vi "Set Random Colors.vi"(1 "Instrument Prop In":T1 {"Private"."Offset" format="%^_3e"; "Private"."Scale Factors" format="%^_3e"}) -> (0 "Instrument Prop Out":T1 {"Private"."Offset" format="%^_3e"; "Private"."Scale Factors" format="%^_3e"})   [LabVIEW 2019]
uses:
  Sub Controls/Instrument Properties.ctl
  Sub Controls/Public.ctl
  Sub Controls/Private.ctl
  Sub Controls/Instrument Ref.ctl
  Sub Controls/SystemCheckBox-resize.ctl
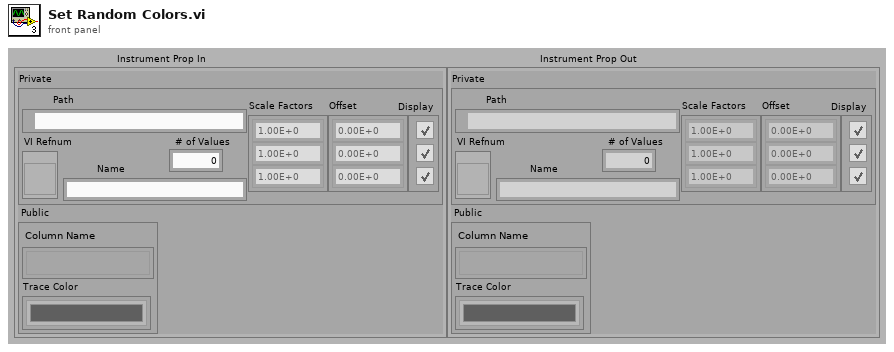
[diagram p1: front panel]
types:
  T1 = typedef "Instrument Properties.ctl" = cluster{"Public":T2, "Private":T3}
  T2 = typedef "Public.ctl" = cluster{"Column Name":string[], "Trace Color":u32[]}
  T3 = typedef "Private.ctl" = cluster{"Path":path, "VI Refnum":T4, "Name":string, "# of Values":i32, "Scale Factors":dbl[], "Display":T5[], "Offset":dbl[]}
  T4 = typedef "Instrument Ref.ctl" = refnum<vi>
  T5 = typedef "SystemCheckBox-resize.ctl" = bool
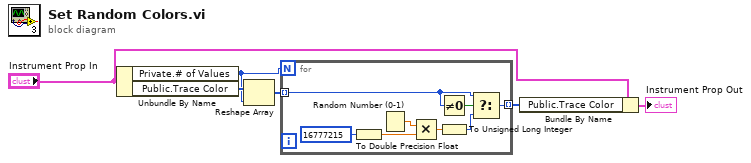
[diagram p0: block diagram]
diagram:
  n1 = Unbundle By Name("Instrument Prop In") -> ("Private.# of Values"=w1:i32, "Public.Trace Color"=w4:u32[])
  n2 = Reshape Array(w4, w1) -> (w2:u32[])
  n3 = for {
    N: w1 -> [_]
    tunnel: w2 -> [w10] mode=indexing
    tunnel: [w9] -> w3 mode=indexing
    n4 = To Double Precision Float(number=u32 16777215 ("y")) -> (double precision float=w7:dbl)
    n5 = Random Number (0-1)() -> (number: 0 to 1=w14:dbl)
    n6 = Multiply(x=w14, y=w7) -> (x*y=w12:dbl)
    n7 = Not Equal To 0?(x=w10) -> (x != 0?=w11:bool)
    n8 = To Unsigned Long Integer(number=w12) -> (unsigned 32bit integer=w8:u32)
    n9 = Select(t=w10, s=w11, f=w8) -> (s? t:f=w9:u32)
  }
  n10 = Bundle By Name(cluster="Instrument Prop In", "Public.Trace Color"=w3) -> (→"Instrument Prop Out":T1)
